vi "uc480_SubVI_Example_Sharpness_Measurement.vi"(8 "Error In":errorcluster, 9 "Measuring Region":u32, 10 "Preset":i32, 11 ".NET (Reference)":refnum<k24>) -> (0 "Error Out":errorcluster, 3 "Sharpness":u32)   [LabVIEW 2011]
uses:
  C:/Program Files/Thorlabs/Scientific Imaging/DCx Camera Support/Develop/DotNet/uc480DotNet.dll
  Develop/DotNet/uc480DotNet.dll
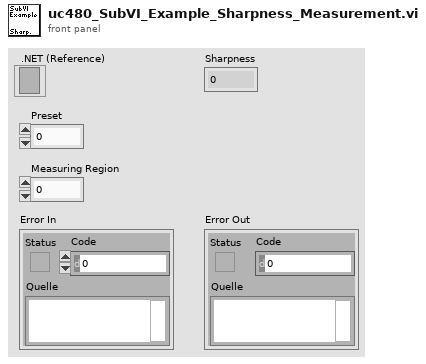
[diagram p1: front panel]
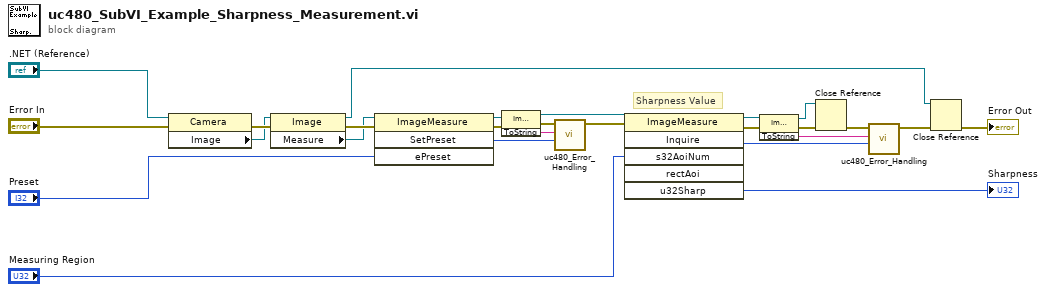
[diagram p0: block diagram]
diagram:
  # "Sharpness Value"
  n1 = property on="Eigenschaftsknoten" class="Camera"(reference=".NET (Reference)", error in="Error In") -> (error out=w15:errorcluster, "Image"=w12:refnum<k24>)  [unwired: 1 out]
  n2 = property on="Eigenschaftsknoten" class="Image"(reference=w12, error in=w15) -> (reference out=w1:refnum<k24>, error out=w16:errorcluster, "Measure"=w13:refnum<k24>)
  n3 = invoke class="ImageMeasure" method="SetPreset"(reference=w13, error in=w16, "ePreset"="Preset") -> (reference out=w21:refnum<k24>, error out=w20:errorcluster, "SetPreset"=w19:i32)  [unwired: 1 in, 1 out]
  n4 = invoke class="ImageMeasure" method="ToString"(reference=w21, error in=w20) -> (reference out=w7:refnum<k24>, error out=w17:errorcluster, "ToString"=w18:string)  [unwired: 1 in]
  n5 = call "uc480_Error_Handling.vi"("Error Code"=w19, "Error String"=w18, "Error In"=w17) -> ("Error Out"=w22:errorcluster)  [unwired: 8 in]
  n6 = invoke class="ImageMeasure" method="Inquire"(reference=w7, error in=w22, "s32AoiNum"="Measuring Region") -> (reference out=w26:refnum<k24>, error out=w25:errorcluster, "Inquire"=w24:i32, "u32Sharp"=→"Sharpness":u32)  [unwired: 3 in, 2 out]
  n7 = invoke class="ImageMeasure" method="ToString"(reference=w26, error in=w25) -> (reference out=w4:refnum<k24>, error out=w6:errorcluster, "ToString"=w23:string)  [unwired: 1 in]
  n8 = Close Reference(reference=w4, error in (no error)=w6) -> (error out=w5:errorcluster)
  n9 = call "uc480_Error_Handling.vi"("Error Code"=w24, "Error String"=w23, "Error In"=w5) -> ("Error Out"=w3:errorcluster)  [unwired: 8 in]
  n10 = Close Reference(reference=w1, error in (no error)=w3) -> (error out=→"Error Out":errorcluster)
